vi "Teleop.vi"(10 "Match Info":T3={"Autonomous Elapsed Seconds"=0.0, "TeleOp Elapsed Seconds"=0.0, "Disabled Elapsed Seconds"=0.0, "Visited Autonomous"=FALSE, "Visited TeleOp"=FALSE, "Visited Disabled"=FALSE, "Autonomous Settings"={"Autonomous Style"=enum."Independent", "VI Refnum"=refnum}}, 11 "Call Context":T4) -> ()   [LabVIEW 2012]
doc: "This VI is called for each TeleOp packet received from the DS where the robot is not disabled. It is often used to read from the joysticks and update I/O or to update setpoints for timed control loops. It should complete and return within 20 milliseconds or it may miss DS packets."
uses:
  <vilib>/Rock Robotics/WPI/DriverStation/WPI_DriverStationDerivedRobotMode.ctl
  <vilib>/Rock Robotics/WPI/DriverStation/WPI_DriverStationMatch Info.ctl
  <vilib>/Rock Robotics/WPI/Joystick/WPI_JoystickButtonState.ctl
  Robot Global Data.vi
  <vilib>/Rock Robotics/WPI/Joystick/WPI_JoystickGetSetRefNum.vi
panel:
  out "turn":dbl
  out "driveRight":dbl
  out "driveLeft":dbl
  out "Steering":dbl(slide) scale=-1.0..1.0
  out "Throttle":dbl(slide) scale=-1.0..1.0
  out "armPower":dbl
  in  "NunchukJoystickIncreaser":dbl=1.5
  out "driverErrorHandler":errorcluster
  out "operatorErrorHandler":errorcluster
  out "nunchukErrorHandler":errorcluster
  out "Nunchuck Axes":T1
  out "Nunchuck Buttons":T2
  out "Operator Buttons":T2
  out "OperatorAxes":T1
  out "Driver Buttons":T2
  out "Driver Axes":T1
  # "DRIVER"
  # "OPERATOR"
  # "NUNCHUCK"
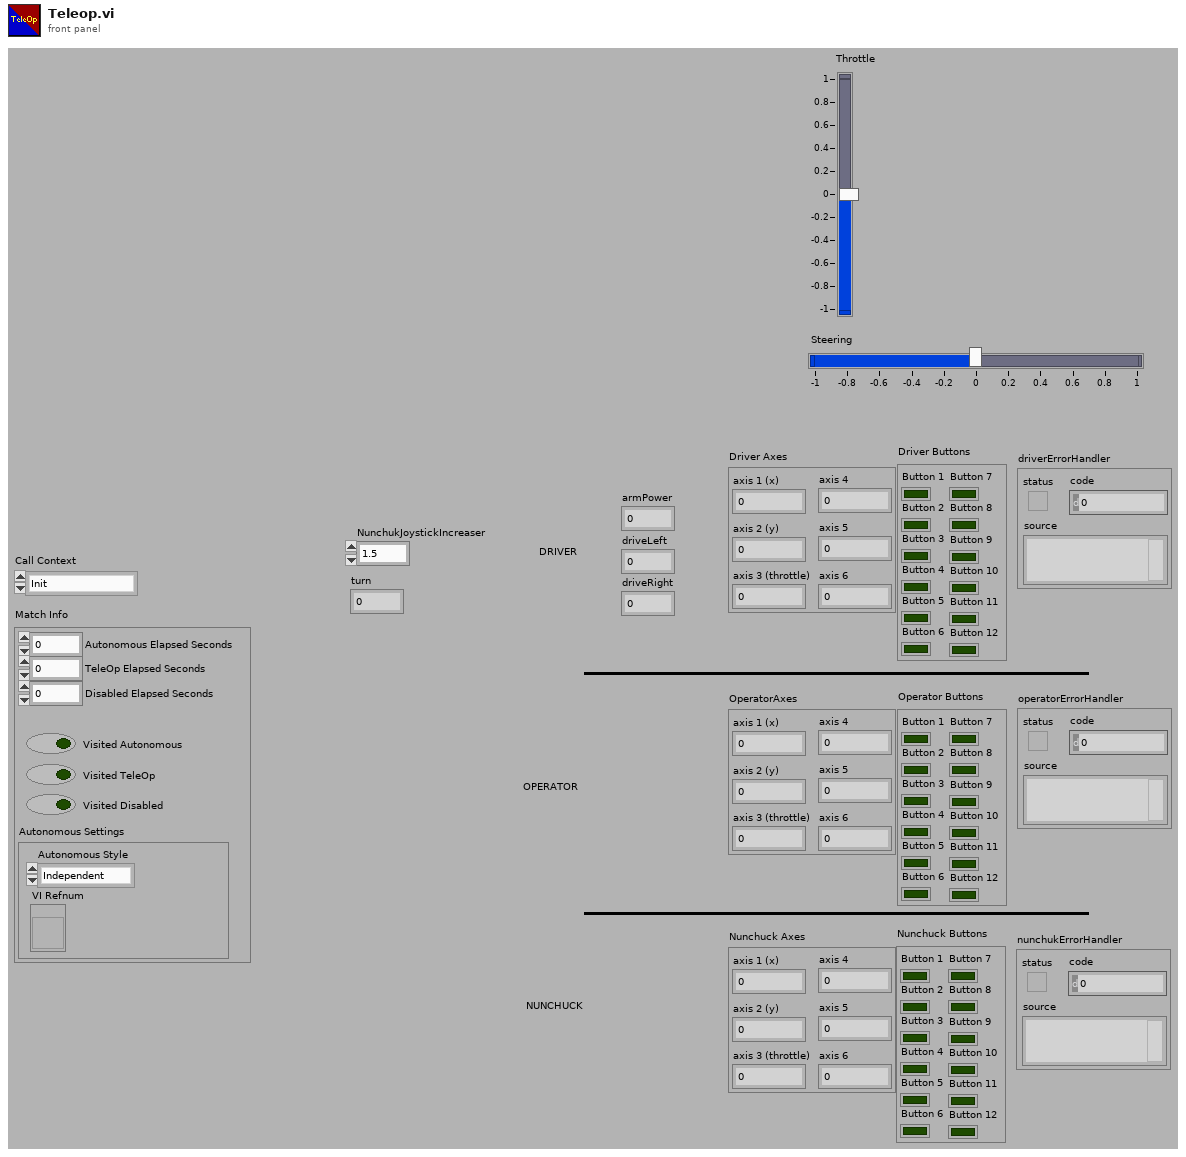
[diagram p1: front panel]
types:
  T1 = cluster{"axis 1 (x)":dbl, "axis 2 (y)":dbl, "axis 3 (throttle)":dbl, "axis 4":dbl, "axis 5":dbl, "axis 6":dbl}
  T2 = typedef "WPI_JoystickButtonState.ctl" = cluster{"Button 1":bool, "Button 2":bool, "Button 3":bool, "Button 4":bool, "Button 5":bool, "Button 6":bool, "Button 7":bool, "Button 8":bool, "Button 9":bool, "Button 10":bool, "Button 11":bool, "Button 12":bool}
  T3 = typedef "WPI_DriverStationMatch Info.ctl" = cluster{"Autonomous Elapsed Seconds":dbl, "TeleOp Elapsed Seconds":dbl, "Disabled Elapsed Seconds":dbl, "Visited Autonomous":bool, "Visited TeleOp":bool, "Visited Disabled":bool, "Autonomous Settings":cluster{"Autonomous Style":enum16{"Iterative", "Independent"}, "VI Refnum":refnum<vi>}}
  T4 = typedef "WPI_DriverStationDerivedRobotMode.ctl" = enum16{"Init", "Execute", "Stop"}
  T5 = typedef "WPI_JoystickDevRef.ctl" = cluster{"Device":T6}
  T6 = typedef "WPI_JoystickDeviceEnum.ctl" = enum16{"USB 1", "USB 2", "USB 3", "USB 4", "Kinect 1", "Kinect 2"}
  T7 = typedef "WPI_AnalogChannelDevRef.ctl" = cluster{"DevStatus":errorcluster, "Analog Module":T8, "Analog Channel":T9}
  T8 = typedef "FPGA_TypedefAnalogModule.ctl" = enum16{"Analog Module 1", "Analog Module 2"}
  T9 = typedef "FPGA_AIChannel.ctl" = enum8{"AI 1", "AI 2", "AI 3", "AI 4", "AI 5", "AI 6", "AI 7", "AI 8", "Invalid"}
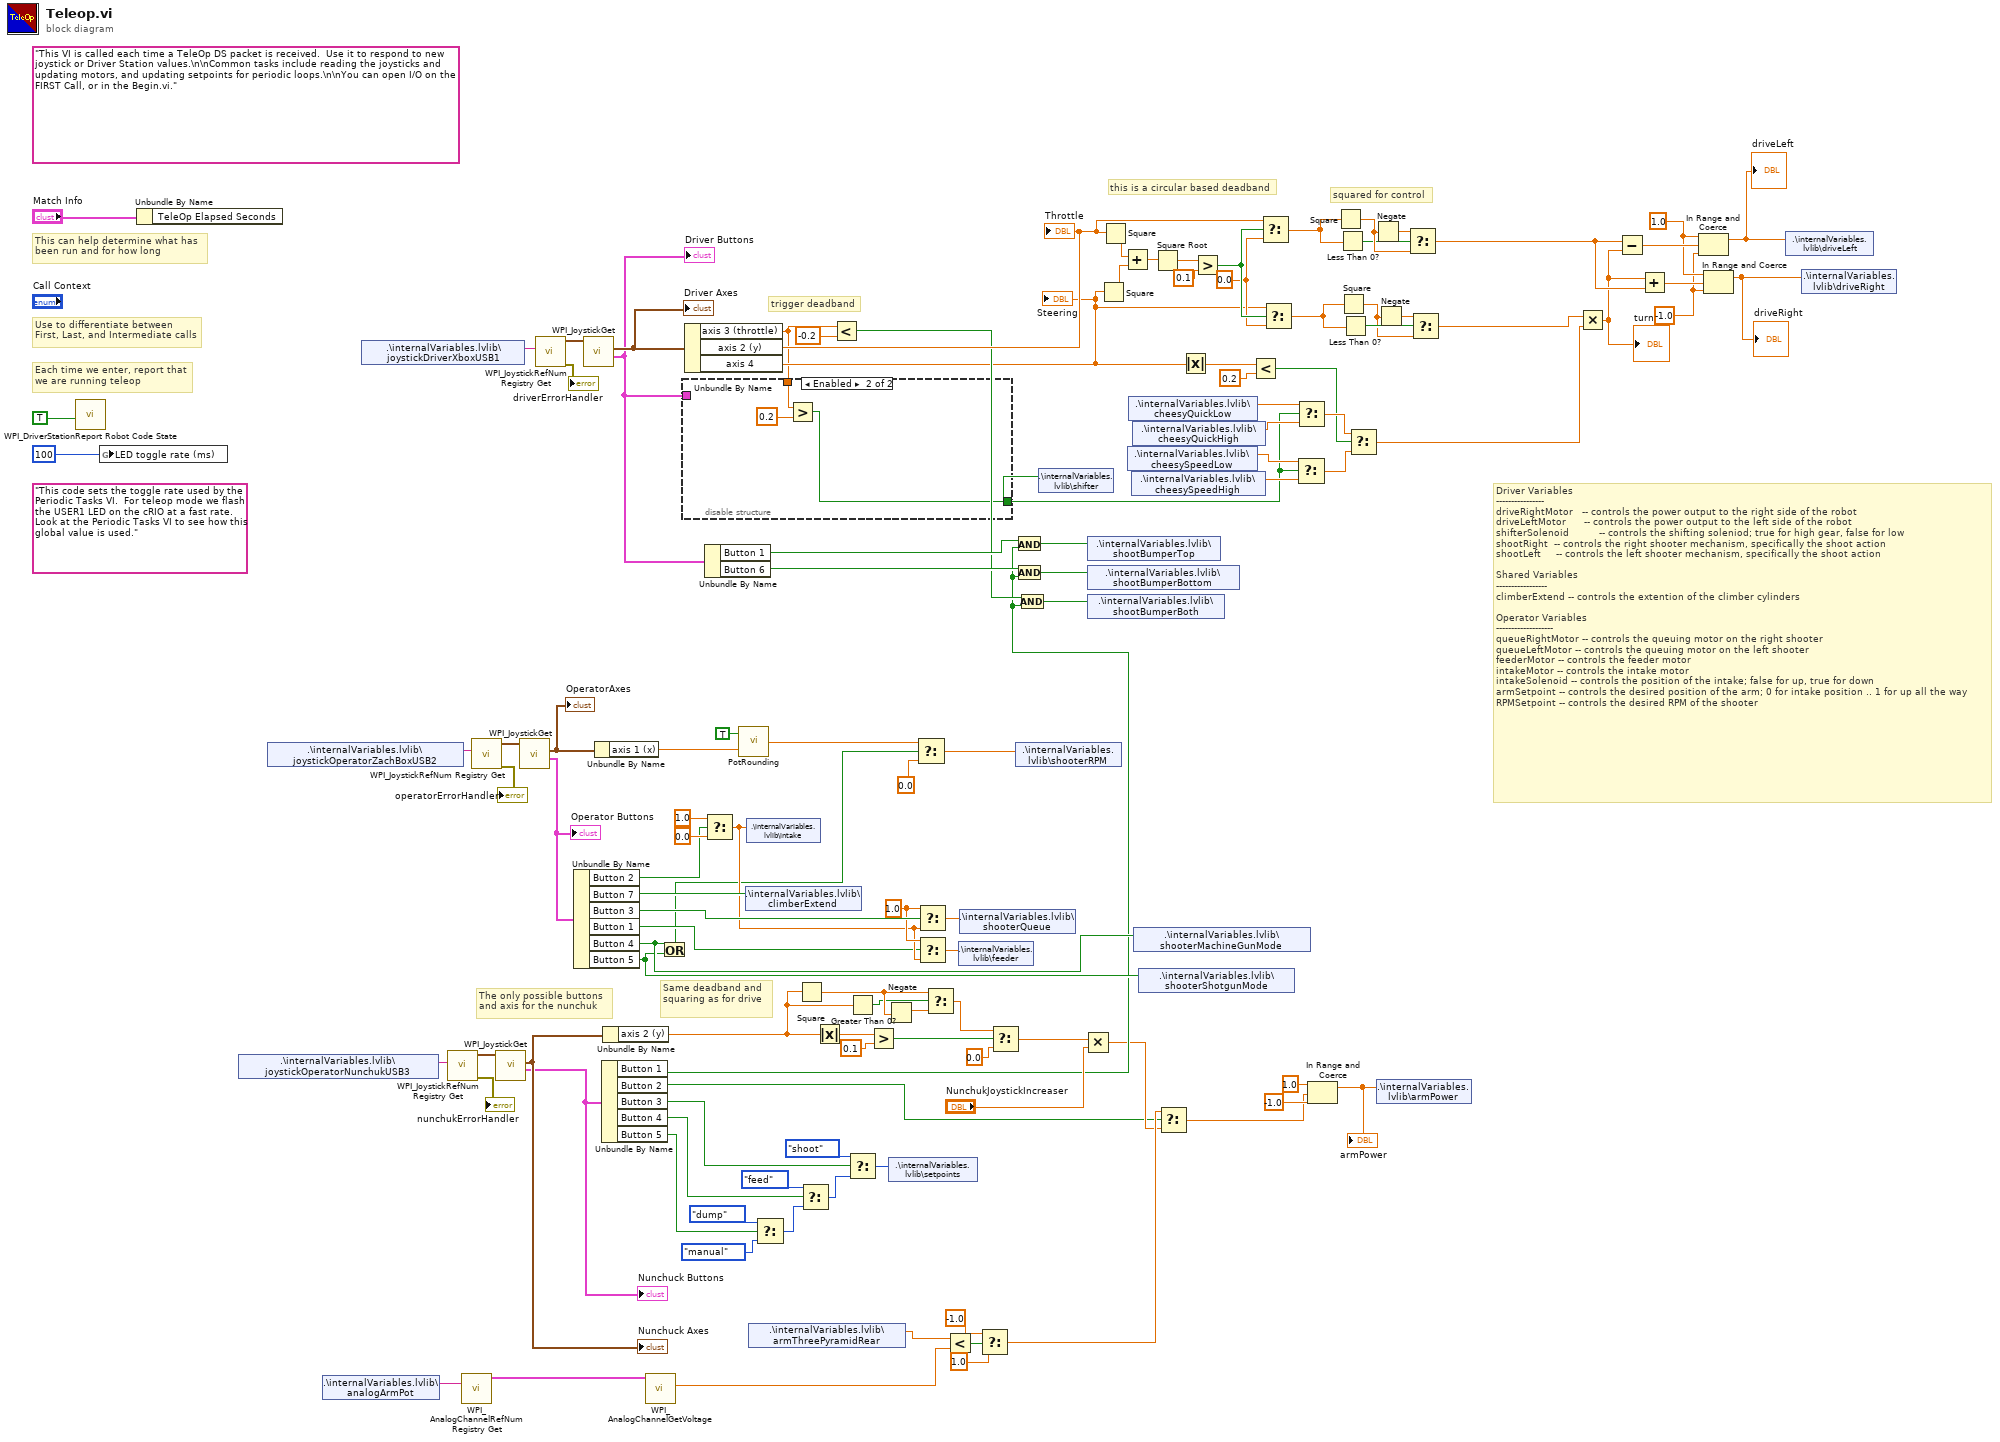
[diagram p0: block diagram]
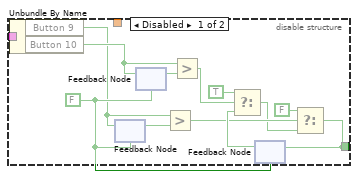
[diagram p2: hidden frame]
diagram:
  w39 = -1.0 ("lower limit")
  w40 = 1.0 ("upper limit")
  w61 = 0.0 ("f")
  w107 = 1.0 ("t")
  (unwired) "This code sets the toggle rate used by the Periodic Tasks VI.  For teleop mode we flash the USER1 LED on the cRIO at a fast rate.  Look at the Periodic Tasks VI to see how this global value is used."
  (unwired) "This VI is called each time a TeleOp DS packet is received.  Use it to respond to new joystick or Driver Station values.\n\nCommon tasks include reading the joysticks and updating motors, and updating setpoints for periodic loops.\n\nYou can open I/O on the FIRST Call, or in the Begin.vi."
  # "squared for control"
  # "this is a circular based deadband"
  # "The only possible buttons and axis for the nunchuk"
  # "Same deadband and squaring as for drive"
  # "Driver Variables\n----------------\ndriveRightMotor   -- controls the power output to the right side of the robot\ndriveLeftMotor      -- controls the power output to the left side of the robot\nshifterSolenoid          -- controls the shifting soleniod; true for high gear, false for low\nshootRight  -- controls the right shooter mechanism, specifically the shoot action\nshootLeft     -- controls the left shooter mechanism, specifically the shoot action\n\nShared Variables\n-----------------\nclimberExtend -- controls the extention of the climber cylinders\n\nOperator Variables\n-------------------\nqueueRightMotor -- controls the queuing motor on the right shooter\nqueueLeftMotor -- controls the queuing motor on the left shooter\nfeederMotor -- controls the feeder motor\nintakeMotor -- controls the intake motor\nintakeSolenoid -- controls the position of the intake; false for up, true for down\narmSetpoint -- controls the desired position of the arm; 0 for intake position .. 1 for up all the way\nRPMSetpoint -- controls the desired RPM of the shooter"
  # "trigger deadband"
  # "Each time we enter, report that\nwe are running teleop"
  # "Use to differentiate between\nFirst, Last, and Intermediate calls"
  # "This can help determine what has\nbeen run and for how long"
  n1 = call <vilib>:"WPI_DriverStationReport Robot Code State.vi"("TeleOp"=TRUE ("Autonomous")) -> ()  [unwired: 10 in, 1 out]
  n2 = global write "Robot Global Data.vi" "LED toggle rate (ms)"(u32 100 ("LED ms toggle rate")) -> ()
  n3 = Unbundle By Name("Match Info") -> ()  [unwired: 1 out]
  n4 = shared-variable ".\\internalVariables.lvlib\\joystickOperatorNunchukUSB3"() -> (w41:string)  [unwired: 1 in, 1 out]
  n5 = shared-variable ".\\internalVariables.lvlib\\joystickOperatorZachBoxUSB2"() -> (w42:string)  [unwired: 1 in, 1 out]
  n6 = shared-variable ".\\internalVariables.lvlib\\analogArmPot"() -> (w21:string)  [unwired: 1 in, 1 out]
  n7 = shared-variable ".\\internalVariables.lvlib\\joystickDriverXboxUSB1"() -> (w43:string)  [unwired: 1 in, 1 out]
  n8 = call <vilib>:"WPI_JoystickRefNum Registry Get.vi"("refnum name"=w41) -> ("error out"=→"nunchukErrorHandler":errorcluster, "JoystickDevRef"=w103:T5)  [unwired: 1 in, 8 out]
  n9 = call <vilib>:"WPI_AnalogChannelRefNum Registry Get.vi"("refnum name"=w21) -> ("AIDeviceRef"=w22:T7)  [unwired: 9 in, 1 out]
  n10 = call <vilib>:"WPI_JoystickRefNum Registry Get.vi"("refnum name"=w42) -> ("error out"=→"operatorErrorHandler":errorcluster, "JoystickDevRef"=w116:T5)  [unwired: 1 in, 8 out]
  n11 = call <vilib>:"WPI_JoystickGet.vi"("JoystickDevRef"=w103) -> ("Buttons"=w101:T2, "Axes"=w102:T1)  [unwired: 1 in, 4 out]
  "Nunchuck Buttons" <- w101
  "Nunchuck Axes" <- w102
  n12 = call <vilib>:"WPI_JoystickGet.vi"("JoystickDevRef"=w116) -> ("Buttons"=w109:T2, "Axes"=w113:T1)  [unwired: 1 in, 4 out]
  "OperatorAxes" <- w113
  "Operator Buttons" <- w109
  n13 = call <vilib>:"WPI_JoystickRefNum Registry Get.vi"("refnum name"=w43) -> ("error out"=→"driverErrorHandler":errorcluster, "JoystickDevRef"=w112:T5)  [unwired: 1 in, 8 out]
  n14 = Unbundle By Name(w109) -> ("Button 2"=w98:bool, "Button 7"=w104:bool, "Button 3"=w108:bool, "Button 1"=w91:bool, "Button 4"=w78:bool, "Button 5"=w77:bool)
  n15 = call <vilib>:"WPI_JoystickGet.vi"("JoystickDevRef"=w112) -> ("Buttons"=w51:T2, "Axes"=w111:T1)  [unwired: 1 in, 4 out]
  "Driver Axes" <- w111
  "Driver Buttons" <- w51
  n16 = Unbundle By Name(w113) -> ("axis 1 (x)"=w96:dbl)
  n17 = Unbundle By Name(w101) -> ("Button 1"=w44:bool, "Button 2"=w12:bool, "Button 3"=w9:bool, "Button 4"=w8:bool, "Button 5"=w7:bool)
  n18 = Unbundle By Name(w102) -> ("axis 2 (y)"=w1:dbl)
  n19 = call <vilib>:"WPI_AnalogChannelGetVoltage.vi"("AIDeviceRef"=w22) -> ("Voltage"=w14:dbl)  [unwired: 8 in, 2 out]
  n20 = Or(x=w78, y=w77) -> (x .or. y?=w82:bool)
  n21 = Unbundle By Name(w111) -> ("axis 3 (throttle)"=w24:dbl, "axis 2 (y)"=w52:dbl, "axis 4"=w26:dbl)
  "Throttle" <- w52
  "Steering" <- w26
  n22 = disable-structure shown="Enabled" {
    disable-tunnel: w51 -> [w121 _]
    disable-tunnel: [w120 w131] -> w28
    disable-tunnel: w24 -> [_ w133]
    frame Disabled {
      w122 = FALSE ("t")
      n23 = Unbundle By Name(w121) -> ("Button 9"=w118:bool, "Button 10"=w119:bool)
      n24 = feedback #1(w122) -> (w129:bool)
      n25 = feedback-in #1(w118) -> ()
      n26 = feedback #2(w122) -> (w130:bool)
      n27 = feedback-in #2(w119) -> ()
      n28 = Greater?(x=w118, y=w129) -> (0:w126:bool)
      n29 = Greater?(x=w119, y=w130) -> (0:w124:bool)
      n30 = feedback #3(w122) -> (w127:bool)
      n31 = Select(t=TRUE, s=w124, f=w127) -> (s? t:f=w125:bool)
      n32 = Select(t=FALSE, s=w126, f=w125) -> (s? t:f=w120:bool)
      n33 = feedback-in #3(w120) -> ()
    }
    frame Enabled {
      n34 = Greater?(x=w133, y=0.2) -> (0:w131:bool)
    }
  }
  n35 = Unbundle By Name(w51) -> ("Button 1"=w75:bool, "Button 6"=w76:bool)
  n36 = Select(t=1.0, s=w98, f=0.0) -> (s? t:f=w97:dbl)
  n37 = call "PotRounding.vi"("Potentiometer"=w96, "Invert?"=TRUE) -> ("shooter output"=w80:dbl)
  n38 = shared-variable ".\\internalVariables.lvlib\\climberExtend"(w104) -> ()  [unwired: 1 in, 1 out]
  n39 = shared-variable ".\\internalVariables.lvlib\\intake"(w97) -> ()  [unwired: 1 in, 1 out]
  n40 = shared-variable ".\\internalVariables.lvlib\\armThreePyramidRear"() -> (w13:dbl)  [unwired: 1 in, 1 out]
  n41 = Select(t=enum16{"manual", "shoot", "feed", "dump"}."dump" ("setpoints"), s=w7, f=enum16{"manual", "shoot", "feed", "dump"}."manual" ("setpoints")) -> (s? t:f=w11:enum16{"manual", "shoot", "feed", "dump"})
  n42 = Square(x=w1) -> (x^2=w89:dbl)
  n43 = Select(t=enum16{"manual", "shoot", "feed", "dump"}."feed" ("setpoints"), s=w8, f=w11) -> (s? t:f=w10:enum16{"manual", "shoot", "feed", "dump"})
  n44 = Absolute Value(x=w1) -> (abs(x)=w94:dbl)
  n45 = Less?(x=w24, y=-0.2) -> (x < y?=w45:bool)
  n46 = Greater Than 0?(x=w1) -> (x > 0?=w88:bool)
  n47 = Select(t=enum16{"manual", "shoot", "feed", "dump"}."shoot" ("setpoints"), s=w9, f=w10) -> (s? t:f=w3:enum16{"manual", "shoot", "feed", "dump"})
  n48 = Greater?(x=w94, y=0.1) -> (0:w93:bool)
  n49 = Negate(x=w89) -> (-x=w90:dbl)
  n50 = shared-variable ".\\internalVariables.lvlib\\setpoints"(w3) -> ()  [unwired: 1 in, 1 out]
  n51 = Select(t=w80, s=w82, f=0.0) -> (s? t:f=w79:dbl)
  n52 = Select(t=w107, s=w108, f=w97) -> (s? t:f=w106:dbl)
  n53 = Select(t=w107, s=w91, f=w97) -> (s? t:f=w105:dbl)
  n54 = Select(t=w89, s=w88, f=w90) -> (s? t:f=w87:dbl)
  n55 = Less?(x=w13, y=w14) -> (x < y?=w20:bool)
  n56 = shared-variable ".\\internalVariables.lvlib\\feeder"(w105) -> ()  [unwired: 1 in, 1 out]
  n57 = shared-variable ".\\internalVariables.lvlib\\shooterQueue"(w106) -> ()  [unwired: 1 in, 1 out]
  n58 = Select(t=-1.0, s=w20, f=1.0) -> (s? t:f=w17:dbl)
  n59 = Select(t=w87, s=w93, f=0.0) -> (s? t:f=w70:dbl)
  n60 = And(x=w75, y=w44) -> (x .and. y?=w74:bool)
  n61 = And(x=w76, y=w44) -> (x .and. y?=w72:bool)
  n62 = shared-variable ".\\internalVariables.lvlib\\shooterRPM"(w79) -> ()  [unwired: 1 in, 1 out]
  n63 = And(x=w45, y=w44) -> (x .and. y?=w73:bool)
  n64 = shared-variable ".\\internalVariables.lvlib\\shifter"(w28) -> ()  [unwired: 1 in, 1 out]
  n65 = Multiply(x=w70, y="NunchukJoystickIncreaser") -> (x*y=w16:dbl)
  n66 = shared-variable ".\\internalVariables.lvlib\\shootBumperTop"(w74) -> ()  [unwired: 1 in, 1 out]
  n67 = shared-variable ".\\internalVariables.lvlib\\shootBumperBottom"(w72) -> ()  [unwired: 1 in, 1 out]
  n68 = shared-variable ".\\internalVariables.lvlib\\shootBumperBoth"(w73) -> ()  [unwired: 1 in, 1 out]
  n69 = Square(x=w26) -> (x^2=w66:dbl)
  n70 = Square(x=w52) -> (x^2=w67:dbl)
  n71 = Add(x=w67, y=w66) -> (x+y=w65:dbl)
  n72 = shared-variable ".\\internalVariables.lvlib\\cheesySpeedLow"() -> (w35:dbl)  [unwired: 1 in, 1 out]
  n73 = shared-variable ".\\internalVariables.lvlib\\cheesyQuickLow"() -> (w33:dbl)  [unwired: 1 in, 1 out]
  n74 = shared-variable ".\\internalVariables.lvlib\\cheesySpeedHigh"() -> (w36:dbl)  [unwired: 1 in, 1 out]
  n75 = shared-variable ".\\internalVariables.lvlib\\cheesyQuickHigh"() -> (w34:dbl)  [unwired: 1 in, 1 out]
  n76 = shared-variable ".\\internalVariables.lvlib\\shooterMachineGunMode"(w78) -> ()  [unwired: 1 in, 1 out]
  n77 = shared-variable ".\\internalVariables.lvlib\\shooterShotgunMode"(w77) -> ()  [unwired: 1 in, 1 out]
  n78 = Square Root(x=w65) -> (sqrt(x)=w64:dbl)
  n79 = Select(t=w17, s=w12, f=w16) -> (s? t:f=w15:dbl)
  n80 = Absolute Value(x=w26) -> (abs(x)=w25:dbl)
  n81 = Greater?(x=w64, y=0.1) -> (0:w62:bool)
  n82 = Less?(x=w25, y=0.2) -> (x < y?=w31:bool)
  n83 = Select(t=w52, s=w62, f=w61) -> (s? t:f=w53:dbl)
  n84 = Select(t=w26, s=w62, f=w61) -> (s? t:f=w60:dbl)
  n85 = Select(t=w35, s=w28, f=w36) -> (s? t:f=w37:dbl)
  n86 = Select(t=w33, s=w28, f=w34) -> (s? t:f=w38:dbl)
  n87 = In Range and Coerce(upper limit=1.0, x=w15, lower limit=-1.0) -> (coerced(x)=w68:dbl)  [unwired: 1 out]
  "armPower" <- w68
  n88 = Square(x=w53) -> (x^2=w55:dbl)
  n89 = Less Than 0?(x=w53) -> (x < 0?=w54:bool)
  n90 = Square(x=w60) -> (x^2=w58:dbl)
  n91 = Less Than 0?(x=w60) -> (x < 0?=w59:bool)
  n92 = Select(t=w38, s=w31, f=w37) -> (s? t:f=w29:dbl)
  n93 = Negate(x=w55) -> (-x=w56:dbl)
  n94 = Negate(x=w58) -> (-x=w57:dbl)
  n95 = shared-variable ".\\internalVariables.lvlib\\armPower"(w68) -> ()  [unwired: 1 in, 1 out]
  n96 = Select(t=w56, s=w54, f=w55) -> (s? t:f=w48:dbl)
  n97 = Select(t=w57, s=w59, f=w58) -> (s? t:f=w27:dbl)
  n98 = Multiply(x=w27, y=w29) -> (x*y=w30:dbl)
  "turn" <- w30
  n99 = Subtract(x=w48, y=w30) -> (x-y=w50:dbl)
  n100 = Add(x=w30, y=w48) -> (x+y=w49:dbl)
  n101 = In Range and Coerce(upper limit=w40, x=w50, lower limit=w39) -> (coerced(x)=w47:dbl)  [unwired: 1 out]
  "driveLeft" <- w47
  n102 = In Range and Coerce(upper limit=w40, x=w49, lower limit=w39) -> (coerced(x)=w46:dbl)  [unwired: 1 out]
  "driveRight" <- w46
  n103 = shared-variable ".\\internalVariables.lvlib\\driveLeft"(w47) -> ()  [unwired: 1 in, 1 out]
  n104 = shared-variable ".\\internalVariables.lvlib\\driveRight"(w46) -> ()  [unwired: 1 in, 1 out]
